vi "FlyWheelSim_Execute.vi"(5 "FlyWheelSim_Model _Params":T7={"DCMOTOR_TYPES"=enum."NEO", "Num Motors"=1, "Gearing"=0.75, "MOI kgm2"=26.0} {"MOI kgm2" format="%#_13g"; "Gearing" format="%#_13g"}, 6 "dT_Seconds":dbl=0.02 format="%#_13g", 7 "FlyWheelSim_Simulation_Params":T1={"Vel Meas Std Dev Rad/Sec"=2.0} {"Vel Meas Std Dev Rad/Sec" format="%#_13g"}, 9 "Battery Volts":dbl=12.0, 11 "Motor Dmd":dbl) -> (0 "Error":bool, 2 "Motor Current":dbl, 3 "Velocity_RPM":dbl, 4 "out FlyWheelSim":T2 {"GearBox"."Jr_KgM2" format="%13.5p"; "GearBox"."L_H" format="%13.5p"; "GearBox"."Kt_NMPerAmp" format="%13.5p"; "GearBox"."KvINV_RadPerSecPerVolt" format="%13.5p"; "GearBox"."R_Ohms" format="%13.5p"; "GearBox"."FreeSpeed_RadPerSec" format="%13.5p"; "GearBox"."FreeCurrent_Amps" format="%13.5p"; "GearBox"."StallCurrent_Amps" format="%13.5p"; "GearBox"."StallTorque_NM" format="%13.5p"; "GearBox"."nominalVoltage_Volts" format="%13.5p"})   [LabVIEW 2019, in "Trajectory_Library.lvlib"]
doc: "Single call LabVIEW function to simulate a Flywheel system. \n\nThe flywheel linear system definition is:\n - States\n - angular velocity (Rad/Sec)\n - Inputs:\n - motor voltage\n - Outputs:\n - angular velocity (rad/sec)\n\n\nInputs:\n - LinearSystem Flywheel Model Params -- cluster -- Contains physical configuration for Flywheel system.\n - Flywheel Sim Simulation Params -- cluster -- Contains siulation configuration.\n - Motor Dmd (CO) -- double -- motor demand value (+/- 1.0 )\n - Battery Voltage -- double -- Current simulated battery voltage (Volts)\n - dT Sec -- double -- Update period (Seconds, Default: 0.02)\n\nOutputs:\n - Velocity RPM -- double -- Current flywheel velocity (RPM)\n - Motor Current -- double -- Current motor current (Amps)\n - Error -- boolean -- If TRUE an error occured.\n - outFlyWheelSim -- cluster -- Current internal data cluster."
uses:
  Trajectory_Library.lvlib
  <vilib>/Analysis/Matrix/Datatypes/RealMatrix.ctl
  <vilib>/Analysis/Matrix/NI_Matrix.lvlib
  TypeDef/LINEAR_SYSTEM.ctl
  Enum/DCMOTOR_TYPES_ENUM.ctl
  TypeDef/LINEAR_SYSTEM_SIM.ctl
  TypeDef/DCMOTOR.CTL
  TypeDef/FLYWHEEL_SIM.ctl
  TypeDef/LINEAR_SYSTEM_ID_FLYWHEEL_MODEL.ctl
  TypeDef/FLYWHEEL_SIM_SIMULATION_PARAMS.ctl
panel:
  # "<States, 1>"
  # "<Outputs, 1>"
  # "<Inputs, 1>"
  # "<Outputs, 1>"
  # "<States,States>"
  # "<States,Inputs>"
  # "<Outputs,States>"
  # "<Outputs,Inputs>"
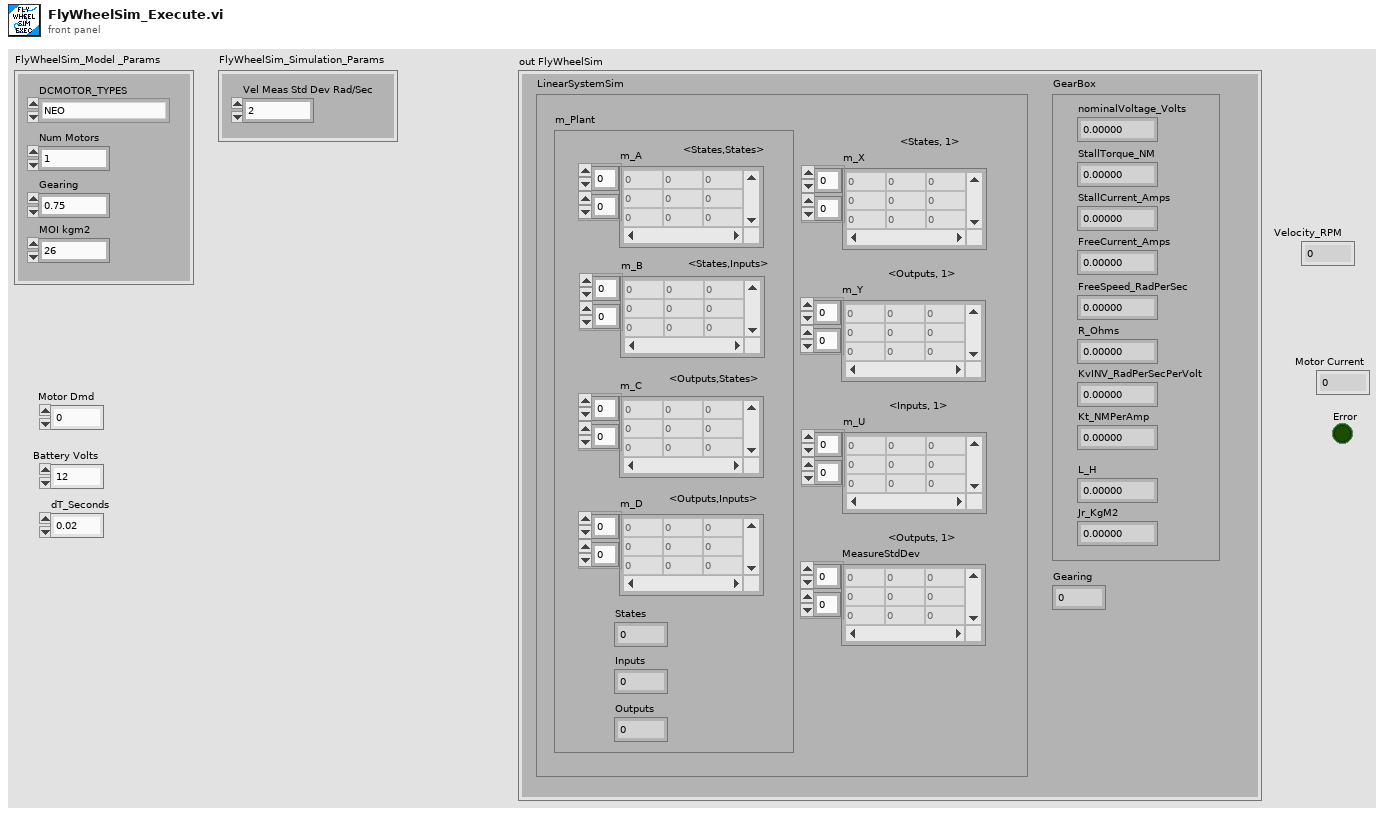
[diagram p1: front panel]
types:
  T1 = typedef "Trajectory_Library.lvlib/FLYWHEEL_SIM_SIMULATION_PARAMS.ctl" = cluster{"Vel Meas Std Dev Rad/Sec":dbl}
  T2 = typedef "Trajectory_Library.lvlib/FLYWHEEL_SIM.ctl" = cluster{"LinearSystemSim":T3, "GearBox":T6, "Gearing":dbl}
  T3 = typedef "Trajectory_Library.lvlib/LINEAR_SYSTEM_SIM.ctl" = cluster{"m_Plant":T4, "m_X":T5, "m_Y":T5, "m_U":T5, "MeasureStdDev":T5}
  T4 = typedef "Trajectory_Library.lvlib/LINEAR_SYSTEM.ctl" = cluster{"m_A":T5, "m_B":T5, "m_C":T5, "m_D":T5, "States":i32, "Inputs":i32, "Outputs":i32}
  T5 = typedef "NI_Matrix.lvlib/RealMatrix.ctl" = dbl[][]
  T6 = typedef "Trajectory_Library.lvlib/DCMOTOR.CTL" = cluster{"nominalVoltage_Volts":dbl, "StallTorque_NM":dbl, "StallCurrent_Amps":dbl, "FreeCurrent_Amps":dbl, "FreeSpeed_RadPerSec":dbl, "R_Ohms":dbl, "KvINV_RadPerSecPerVolt":dbl, "Kt_NMPerAmp":dbl, "L_H":dbl, "Jr_KgM2":dbl}
  T7 = typedef "Trajectory_Library.lvlib/LINEAR_SYSTEM_ID_FLYWHEEL_MODEL.ctl" = cluster{"DCMOTOR_TYPES":T8, "Num Motors":i32, "Gearing":dbl, "MOI kgm2":dbl}
  T8 = typedef "Trajectory_Library.lvlib/DCMOTOR_TYPES_ENUM.ctl" = enum16{"CIM", "AndyMark 9015", "Andy Mark RS 775 125", "Bag", "BaneBots RS 550", "BaneBots RS 775", "Falcon 500", "Mini CIM", "NEO", "NEO 550", "Romi BuiltIn", "Vex 775 Pro", "Snow Blower AM 2235A", "Bosch Seat AM 3493", "Falcon 500 FOC", "Kraken X60", "Kraken X60 FOC", "NEO Vortex"}
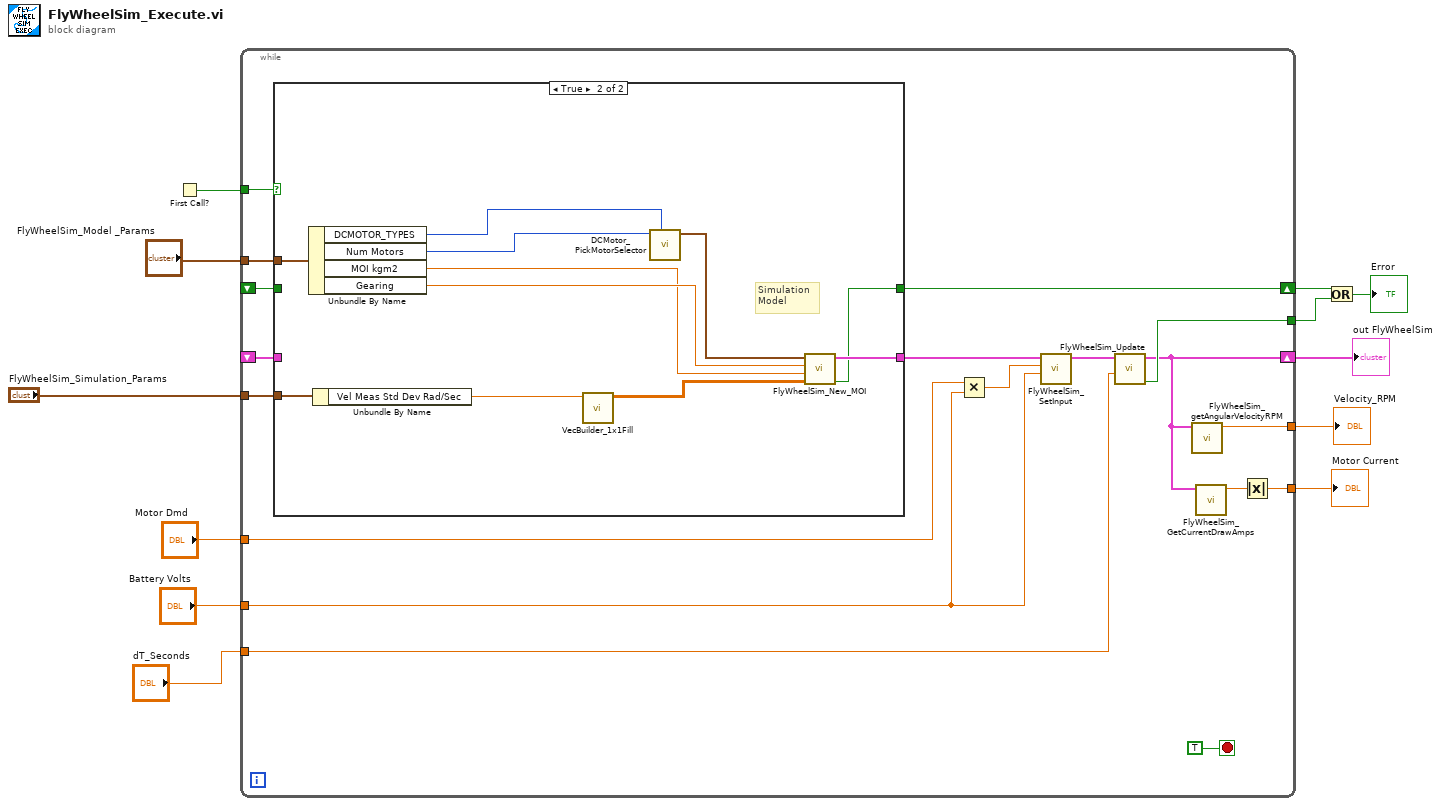
[diagram p0: block diagram]
diagram:
  n1 = First Call?() -> (First Call?: T/F=w11:bool)
  n2 = while {
    tunnel: "FlyWheelSim_Model _Params" -> [w30]
    tunnel: w11 -> [w29]
    shift-right: [w14] -> w2
    shift-left: _ -> [w28]
    shift-right: [w27] -> w6
    shift-left: _ -> [w26]
    tunnel: "Motor Dmd" -> [w22]
    tunnel: "Battery Volts" -> [w21]
    tunnel: [w20] -> w8
    tunnel: [w18] -> w7
    tunnel: [w17] -> w5
    tunnel: "dT_Seconds" -> [w16]
    tunnel: "FlyWheelSim_Simulation_Params" -> [w13]
    stop <- TRUE stop-if-true
    n3 = case shown="True" w29 {
      tunnel: w30 -> [_ w41]
      tunnel: w28 -> [w31 _]
      tunnel: [w32 w35] -> w27
      tunnel: w26 -> [w32 _]
      tunnel: [w31 w36] -> w15
      tunnel: w13 -> [_ w34]
      frame False {
      }
      frame True {
        # "Simulation \nModel"
        n4 = Unbundle By Name(w41) -> ("DCMOTOR_TYPES"=w38:T8, "Num Motors"=w39:i32, "MOI kgm2"=w37:dbl, "Gearing"=w40:dbl)
        n5 = Unbundle By Name(w34) -> ("Vel Meas Std Dev Rad/Sec"=w33:dbl)
        n6 = call "VecBuilder_1x1Fill.vi"("R0_C0"=w33) -> ("output matrix"=w43:T5)  [unwired: 10 in]
        n7 = call "DCMotor_PickMotorSelector.vi"("DCMOTOR_TYPES"=w38, "Num Motors"=w39) -> ("DCMOTOR"=w42:T6)  [unwired: 9 in]
        n8 = call "FlyWheelSim_New_MOI.vi"("MeasurementStdDev"=w43, "jKgMetersSquared"=w37, "Gearing"=w40, "GearBox"=w42) -> ("Error"=w35:bool, "FlyWheelSim"=w36:T2)  [unwired: 6 in]
      }
    }
    n9 = Multiply(x=w22, y=w21) -> (x*y=w25:dbl)
    n10 = call "FlyWheelSim_SetInput.vi"("Battery_Volts"=w21, "Volts"=w25, "FlyWheelSim"=w15) -> ("out FlyWheelSim"=w23:T2)  [unwired: 8 in]
    n11 = call "FlyWheelSim_Update.vi"("dT_Seconds"=w16, "FlyWheelSim"=w23) -> ("Error"=w17:bool, "out FlyWheelSim"=w14:T2)  [unwired: 8 in]
    n12 = call "FlyWheelSim_getAngularVelocityRPM.vi"("FlyWheelSim"=w14) -> ("Velocity_RPM"=w18:dbl)  [unwired: 10 in]
    n13 = call "FlyWheelSim_GetCurrentDrawAmps.vi"("FlyWheelSim"=w14) -> ("Current_Amps"=w24:dbl)  [unwired: 10 in]
    n14 = Absolute Value(x=w24) -> (abs(x)=w20:dbl)
  }
  "Motor Current" <- w8
  "Velocity_RPM" <- w7
  "out FlyWheelSim" <- w2
  n15 = Or(x=w6, y=w5) -> (x .or. y?=→"Error":bool)
